vi "set_P.vi"(8 "error in (no error)":errorcluster, 10 "P":dbl, 11 "connection ID":refnum<k5>) -> (0 "error out":errorcluster, 3 "connection ID out":refnum<k5>)   [LabVIEW 2018]
panel:
  out "bytes written":i32
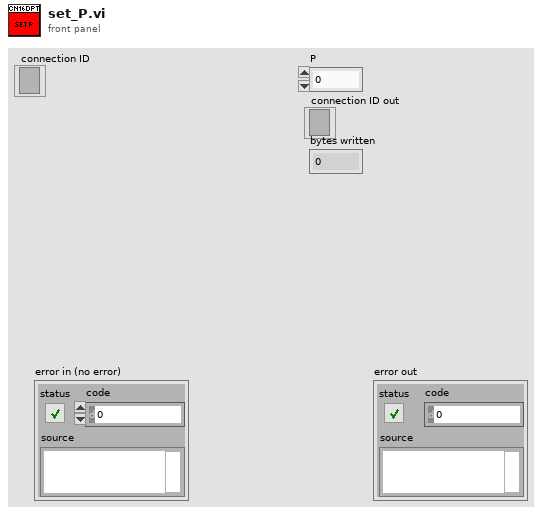
[diagram p1: front panel]
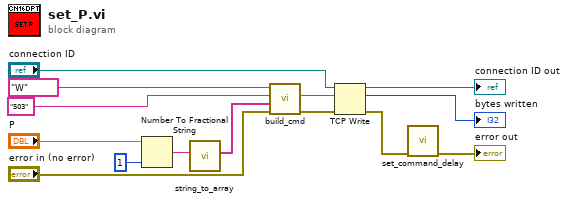
[diagram p0: block diagram]
diagram:
  n1 = Number To Fractional String(number="P", precision (6)=i16 1) -> (F-format string=w7:string)  [unwired: 2 in]
  n2 = call "string_to_array.vi"("String"=w7) -> ("Array"=w6:string[])  [unwired: 10 in]
  n3 = call "build_cmd.vi"("error in (no error)"="error in (no error)", "Parameter list"=w6, "Command ID"="503", "Command class"="W") -> ("error out"=w11:errorcluster, "Command"=w10:string)  [unwired: 6 in]
  n4 = TCP Write(connection ID="connection ID", data in=w10, error in (no error)=w11) -> (connection ID out=→"connection ID out":refnum<k5>, bytes written=→"bytes written":i32, error out=w2:errorcluster)  [unwired: 1 in]
  n5 = call "set_command_delay.vi"("error in (no error)"=w2) -> ("error out"=→"error out":errorcluster)  [unwired: 10 in]
